vi "Load Hardware.vi"(8 "error in (no error)":errorcluster, 10 "Program only changes":bool=TRUE, 11 "Arduino in":refnum<class "Arduino.lvclass">) -> (0 "error out":errorcluster, 3 "Arduino out":refnum<class "Arduino.lvclass">)   [LabVIEW 2013, in "Arduino.lvclass"]
uses:
  Arduino.lvclass
  <vilib>/Instr/_visa.llb/Select Event Type.ctl
  Arduino.lvclass/Arduino.ctl
  <vilib>/Instr/_visa.llb/VISA Configure Serial Port (Serial Instr).vi
panel:
  out "read buffer 2":string
  out "read buffer":string
  # "encapsulate HWI in cluser so each \"last encountered\"\ncan be a different length."
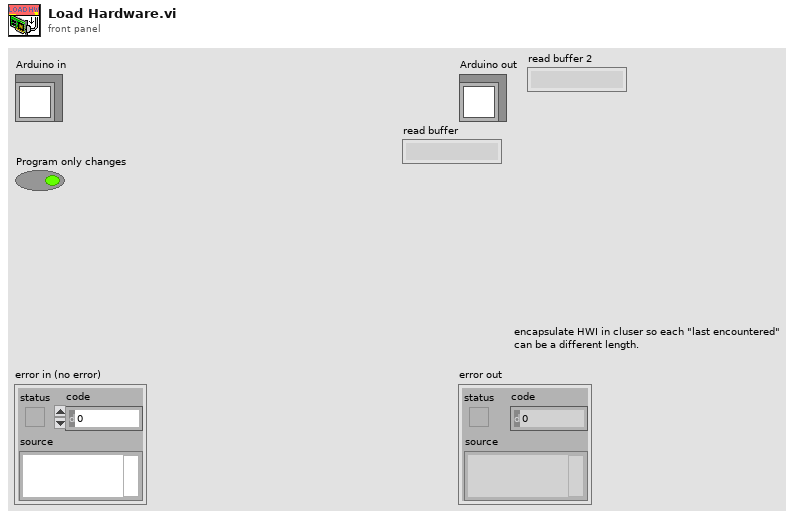
[diagram p1: front panel]
types:
  T1 = typedef "Select Event Type.ctl" = u32
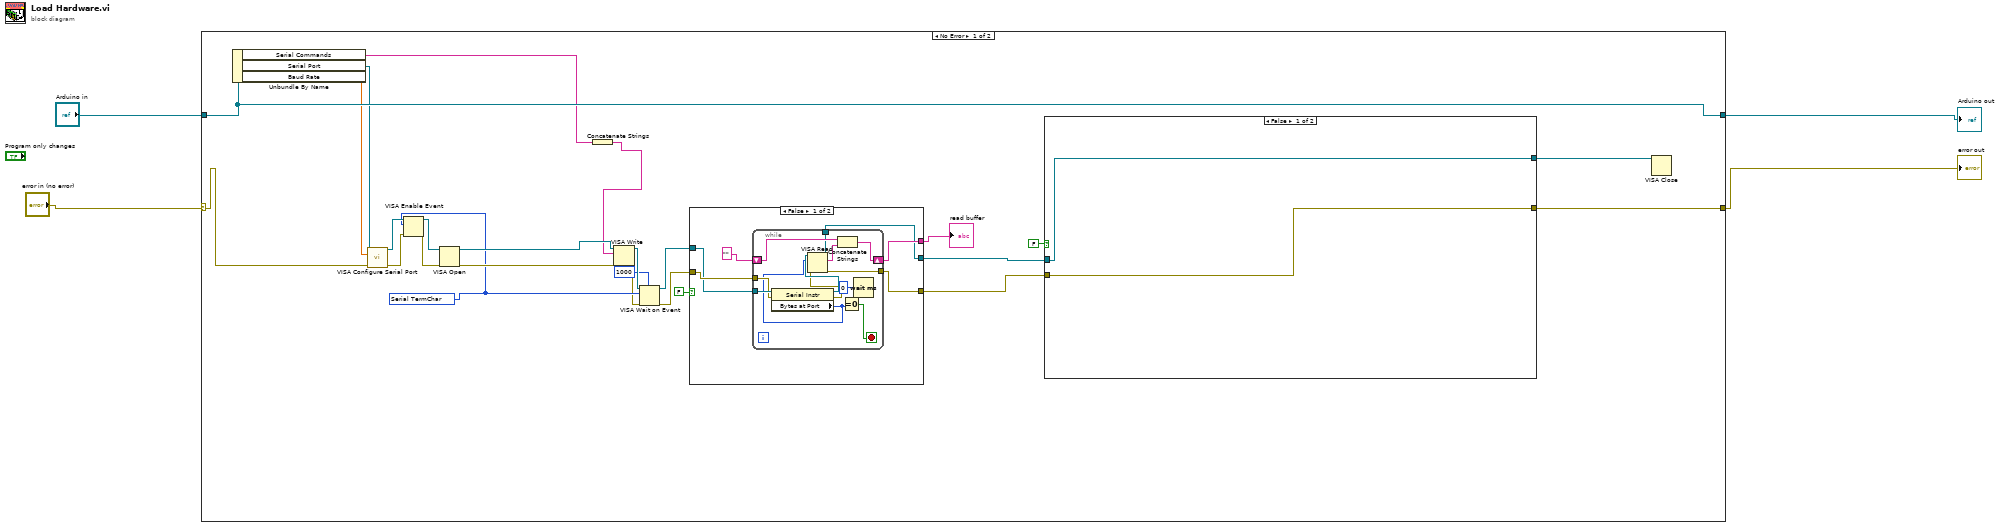
[diagram p0: block diagram]
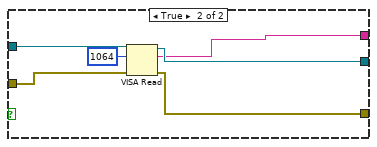
[diagram p2: hidden frame]
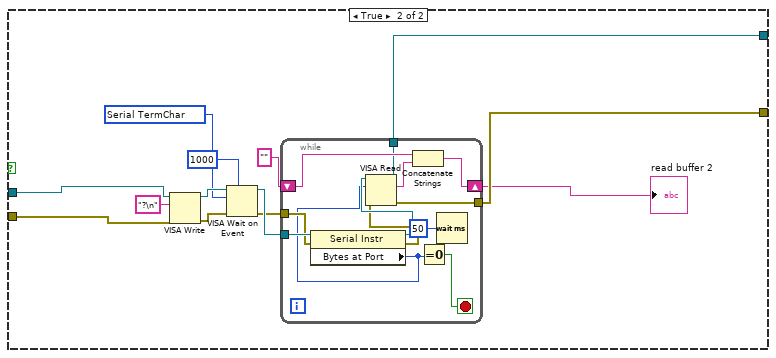
[diagram p3: hidden frame]
diagram:
  n1 = case shown="No Error" "error in (no error)" {
    selector: "error in (no error)" -> [w27 w82]
    tunnel: [w16 w82] -> w1
    tunnel: [w29 w81] -> w3
    tunnel: "Arduino in" -> [w29 w81]
    frame No Error {
      w19 = T1 1073684516 items=["Service Request"=1073684491, "Trigger"=3221168138, "Clear"=1073684493, "VXI Signal"=1073684512, "VXI/VME Interrupt"=3221168161, "VXI/VME Sysfail"=1073684509, "VXI/VME Sysreset"=1073684510, "GPIB CIC"=1073684498, "GPIB Talk"=1073684499, "GPIB Listen"=1073684500, "PXI Interrupt"=1073684514, "Serial Break"=1073684515, "Serial TermChar"=1073684516, "Serial CTS"=1073684521, "Serial DSR"=1073684522, "Serial DCD"=1073684524, "Serial RI"=1073684526, "Serial Character"=1073684533, "USB Interrupt"=1073684535, "All Enabled"=1073709055] ("Event Type")
      n2 = Unbundle By Name(w29) -> ("Serial Commands"=w6:string[], "Serial Port"=w26:refnum<visa-resource-name>, "Baud Rate"=w28:dbl)
      n3 = call-poly "VISA Configure Serial Port"("VISA resource name"=w26, "baud rate (9600)"=w28, "error in (no error)"=w27) -> ("VISA resource name out"=w23:refnum<visa-resource-name>, "error out"=w21:errorcluster)  [unwired: 11 in]
      n4 = VISA Enable Event(8:w21, 10:w19, 11:w23) -> (0:w20:errorcluster, 3:w22:refnum<visa-resource-name>)  [unwired: 1 in]
      n5 = VISA Open(error in (no error)=w20, VISA resource name=w22) -> (VISA resource name=w25:refnum<visa-resource-name>, error out=w24:errorcluster)  [unwired: 3 in]
      n6 = Concatenate Strings(w6) -> (w5:string)
      n7 = VISA Write(VISA resource name=w25, write buffer=w5, error in (no error)=w24) -> (VISA resource name out=w11:refnum<visa-resource-name>, error out=w10:errorcluster)  [unwired: 1 out]
      n8 = VISA Wait on Event(7:u32 1000 ("timeout (0)"), 8:w10, 10:w19, 11:w11) -> (0:w13:errorcluster, 3:w12:refnum<visa-resource-name>)  [unwired: 1 in, 2 out]
      n9 = case shown="False" FALSE {
        tunnel: w13 -> [w31 w53]
        tunnel: w12 -> [w30 w52]
        tunnel: [w32 w51] -> w17
        tunnel: [w33 w50] -> w18
        tunnel: [w34 w48] -> w7
        frame False {
          n10 = while {
            tunnel: w30 -> [w47]
            shift-right: [w43] -> w34
            shift-left: "" ("read buffer") -> [w45]
            tunnel: w31 -> [w41]
            tunnel: [w39] -> w32
            tunnel: [w38] -> w33
            stop <- w46 stop-if-true
            n11 = property class="Serial Instr"(reference=w47, error in=w41) -> (reference out=w42:refnum<visa-resource-name>, error out=w40:errorcluster, "Bytes at Port"=w37:u32)
            n12 = VISA Read(VISA resource name=w42, byte count=w37, error in (no error)=w40) -> (VISA resource name out=w38:refnum<visa-resource-name>, read buffer=w44:string, error out=w39:errorcluster)  [unwired: 1 out]
            n13 = Concatenate Strings(w45, w44) -> (w43:string)
            n14 = Equal To 0?(x=w37) -> (x = 0?=w46:bool)
            n15 = Wait (ms)(milliseconds to wait=u32 0) -> ()  [unwired: 1 out]
          }
        }
        frame True {
          n16 = VISA Read(VISA resource name=w52, byte count=u32 1064, error in (no error)=w53) -> (VISA resource name out=w50:refnum<visa-resource-name>, read buffer=w48:string, error out=w51:errorcluster)  [unwired: 1 out]
        }
      }
      "read buffer" <- w7
      n17 = case shown="False" FALSE {
        tunnel: w18 -> [w55 w67]
        tunnel: w17 -> [w54 w66]
        tunnel: [w54 w59] -> w16
        tunnel: [w55 w58] -> w15
        frame False {
        }
        frame True {
          w63 = T1 1073684516 items=["Service Request"=1073684491, "Trigger"=3221168138, "Clear"=1073684493, "VXI Signal"=1073684512, "VXI/VME Interrupt"=3221168161, "VXI/VME Sysfail"=1073684509, "VXI/VME Sysreset"=1073684510, "GPIB CIC"=1073684498, "GPIB Talk"=1073684499, "GPIB Listen"=1073684500, "PXI Interrupt"=1073684514, "Serial Break"=1073684515, "Serial TermChar"=1073684516, "Serial CTS"=1073684521, "Serial DSR"=1073684522, "Serial DCD"=1073684524, "Serial RI"=1073684526, "Serial Character"=1073684533, "USB Interrupt"=1073684535, "All Enabled"=1073709055] ("Event Type")
          n18 = VISA Write(VISA resource name=w67, write buffer="?\n", error in (no error)=w66) -> (VISA resource name out=w64:refnum<visa-resource-name>, error out=w65:errorcluster)  [unwired: 1 out]
          n19 = VISA Wait on Event(7:u32 1000 ("timeout (0)"), 8:w65, 10:w63, 11:w64) -> (0:w60:errorcluster, 3:w62:refnum<visa-resource-name>)  [unwired: 1 in, 2 out]
          n20 = while {
            tunnel: w62 -> [w80]
            shift-right: [w76] -> w57
            shift-left: "" ("read buffer") -> [w78]
            tunnel: w60 -> [w74]
            tunnel: [w72] -> w59
            tunnel: [w71] -> w58
            stop <- w79 stop-if-true
            n21 = property class="Serial Instr"(reference=w80, error in=w74) -> (reference out=w75:refnum<visa-resource-name>, error out=w73:errorcluster, "Bytes at Port"=w70:u32)
            n22 = VISA Read(VISA resource name=w75, byte count=w70, error in (no error)=w73) -> (VISA resource name out=w71:refnum<visa-resource-name>, read buffer=w77:string, error out=w72:errorcluster)  [unwired: 1 out]
            n23 = Concatenate Strings(w78, w77) -> (w76:string)
            n24 = Equal To 0?(x=w70) -> (x = 0?=w79:bool)
            n25 = Wait (ms)(milliseconds to wait=u32 50) -> ()  [unwired: 1 out]
          }
          "read buffer 2" <- w57
        }
      }
      n26 = VISA Close(VISA resource name=w15) -> ()  [unwired: 1 in, 1 out]
    }
    frame Error {
    }
  }
  "error out" <- w1
  "Arduino out" <- w3
